vi "Parse Single Property.vi"(11 "String In":string) -> (1 "Remaining":string, 2 "Value":string, 3 "Key":string, 5 "JSON Item Type":T1)   [LabVIEW 2020, in "JSON.lvlib"]
doc: "Parses a single property from the string input and can be used to successfully separate properties of an object."
uses:
  JSON.lvlib
  <vilib>/regexp/Match Regular Expression.xnode
  JSON Item Type.ctl
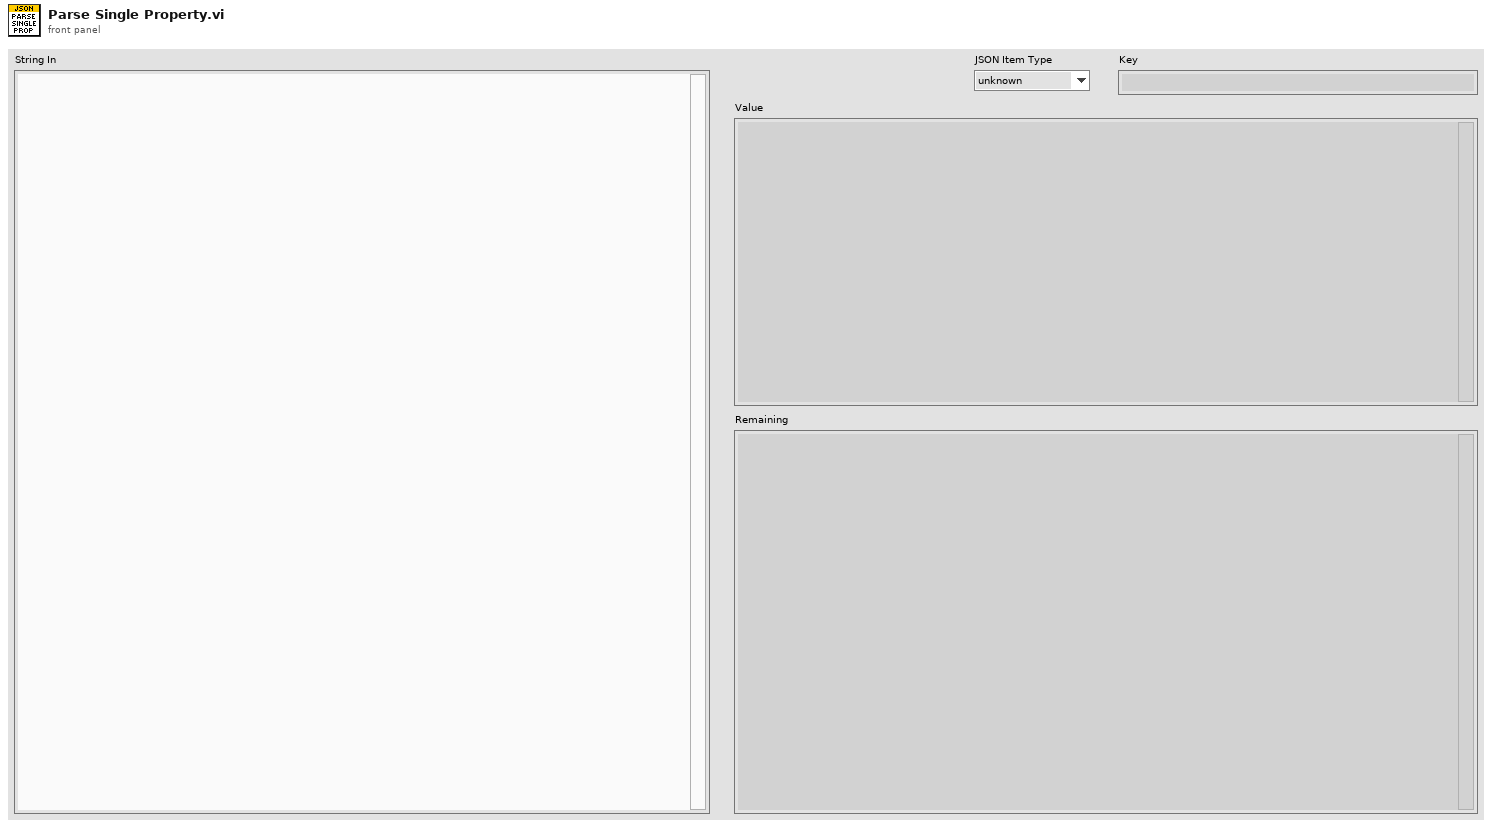
[diagram p1: front panel]
types:
  T1 = typedef "JSON.lvlib/JSON Item Type.ctl" = enum16{"unknown", "null", "Array", "Object", "String", "Number", "Boolean"}
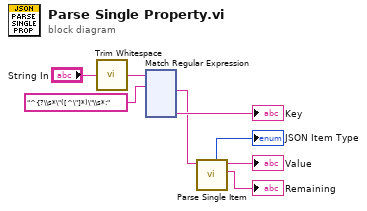
[diagram p0: block diagram]
diagram:
  n1 = call <vilib>:"Trim Whitespace.vi"("string"="String In") -> ("trimmed string"=w7:string)  [unwired: 1 in]
  n2 = xnode "Match Regular Expression"("input string"=w7, "regular expression"="^{?\\s*\"([^\"]*)\"\\s*:") -> ("after match"=w4:string, "submatch 1"=→"Key":string)  [unwired: 4 in, 4 out]
  n3 = call "Parse Single Item.vi"("String In"=w4) -> ("Remaining"=→"Remaining":string, "Item"=→"Value":string, "JSON Item Type"=→"JSON Item Type":T1)  [unwired: 8 in]
